vi "valveDataProc.vi"(0 "frame":u8[](array[numeric])) -> ()   [LabVIEW 2021]
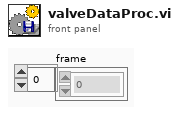
[diagram p1: front panel]
types:
  T1 = cluster{"ValvePos1":sgl, "ValvePos2":sgl, "PressureArray":sgl[], "TempArray2":sgl[], "TempArray1":sgl[], "Valve 1 Time Stamp":timestamp, "Temp 2 Array Time Stamp":timestamp[], "Temp 1 Array Time Stamp":timestamp[], "Valve 2 Time Stamp":timestamp, "Press Array Time Stamp":timestamp[]}
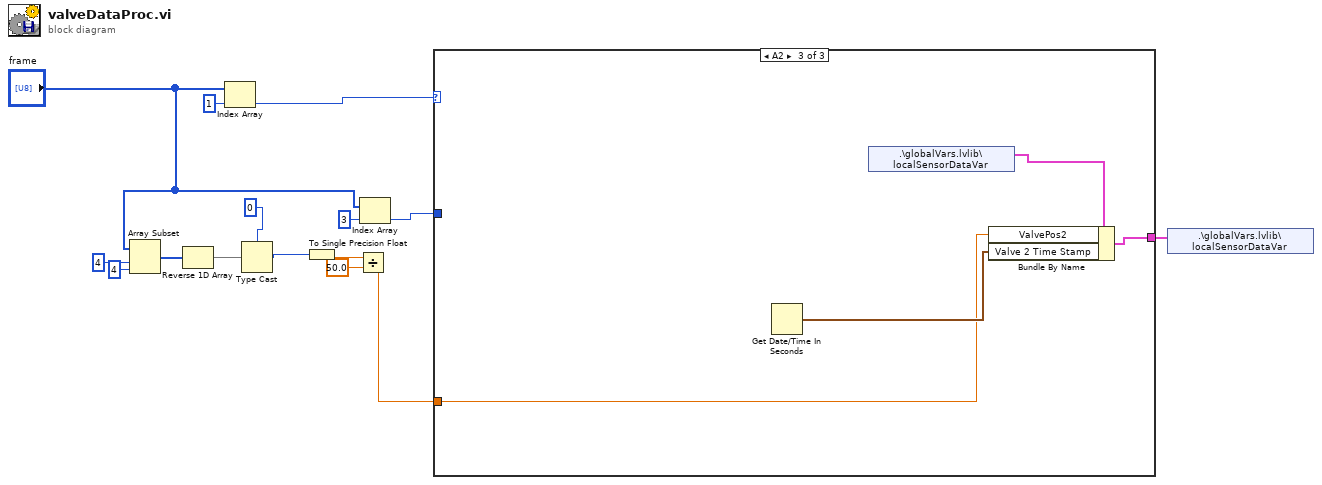
[diagram p0: block diagram]
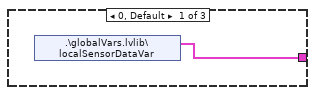
[diagram p2: hidden frame]
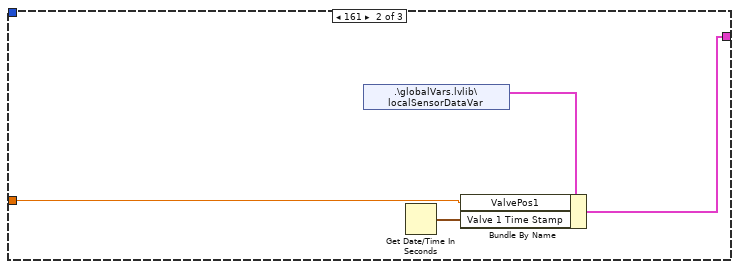
[diagram p3: hidden frame]
diagram:
  n1 = Array Subset(array="frame", index=4, length=4) -> (w7:u8[])
  n2 = Reverse 1D Array(array=w7) -> (reversed array=w6:u8[])
  n3 = Index Array(array="frame", index=1) -> (element=w13:u8)
  n4 = Type Cast(type=0, x=w6) -> (*(type *) &x=w5:i32)
  n5 = To Single Precision Float(number=w5) -> (single precision float=w4:sgl)
  n6 = Divide(x=w4, y=sgl 50.0) -> (x/y=w1:sgl)
  n7 = Index Array(array="frame", index=3) -> (element=w11:u8)
  n8 = case shown="A2" w13 {
    tunnel: [w16 w17 w21] -> w14
    tunnel: w1 -> [_ w19 w23]
    tunnel: w11 -> [_ _ _]
    frame 0, Default {
      n9 = shared-variable ".\\globalVars.lvlib\\localSensorDataVar"() -> (w16:T1)  [unwired: 1 in, 1 out]
    }
    frame 161 {
      n10 = shared-variable ".\\globalVars.lvlib\\localSensorDataVar"() -> (w18:T1)  [unwired: 1 in, 1 out]
      n11 = Get Date/Time In Seconds() -> (seconds since 1Jan1904=w20:timestamp)
      n12 = Bundle By Name(cluster=w18, "ValvePos1"=w19, "Valve 1 Time Stamp"=w20) -> (w17:T1)
    }
    frame 162 {
      n13 = Get Date/Time In Seconds() -> (seconds since 1Jan1904=w24:timestamp)
      n14 = shared-variable ".\\globalVars.lvlib\\localSensorDataVar"() -> (w22:T1)  [unwired: 1 in, 1 out]
      n15 = Bundle By Name(cluster=w22, "ValvePos2"=w23, "Valve 2 Time Stamp"=w24) -> (w21:T1)
    }
  }
  n16 = shared-variable ".\\globalVars.lvlib\\localSensorDataVar"(w14) -> ()  [unwired: 1 in, 1 out]
